vi "Module Init.vi"(8 "error in (no error)":errorcluster, 11 "GUI Manager Module in":refnum<class "GUI Manager Module.lvclass">) -> (0 "error out":errorcluster, 3 "GUI Manager Module out":refnum<class "GUI Manager Module.lvclass">)   [LabVIEW 2020, in "VolatusGUI.lvlib" / "GUI Manager Module.lvclass"]
uses:
  GUI Manager Module.lvclass
  C:/dev/lv20CE/relink/lv-volatus/Volatus/Module/Module.lvclass
  GUI Manager Module.lvclass/GUI Manager Module.ctl
  Volatus/Module/Module.lvclass
  lv-userprefs/User Prefs/PrefsDB/PrefsDB.lvclass
  lv-userprefs/User Prefs/Pref Group/Pref Group.lvclass
  C:/dev/lv20CE/relink/lv-volatus/VolatusGUI/GUI Manager Module/GUI Manager Module.lvclass
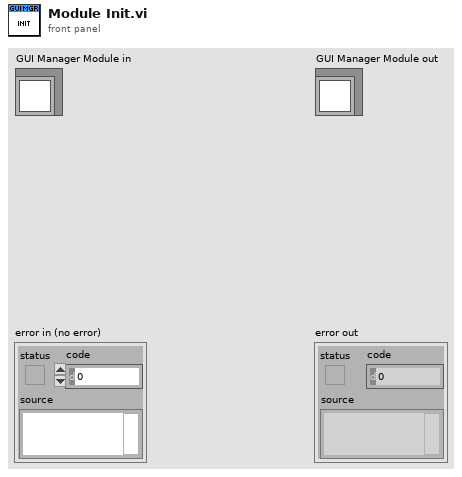
[diagram p1: front panel]
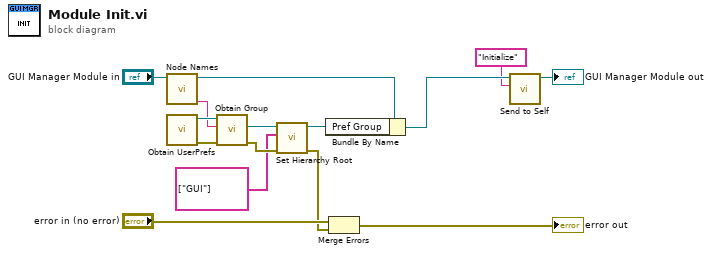
[diagram p0: block diagram]
diagram:
  n1 = call "Node Names.vi"("Module in"="GUI Manager Module in") -> ("Node"=w9:string, "Module out"=w11:refnum<class "GUI Manager Module.lvclass">)  [unwired: 6 in, 3 out]
  n2 = call "Obtain UserPrefs.vi"() -> ("error out"=w14:errorcluster, "PrefsDB out"=w10:refnum<class "PrefsDB.lvclass">)  [unwired: 10 in]
  n3 = call "Obtain Group.vi"("error in (no error)"=w14, "Group"=w9, "PrefsDB in"=w10) -> ("error out"=w15:errorcluster, "Pref Group"=w8:refnum<class "Pref Group.lvclass">)  [unwired: 6 in, 1 out]
  n4 = call "Set Hierarchy Root.vi"("error in (no error)"=w15, "Hierarchy Root"=string[] ["GUI"], "Pref Group in"=w8) -> ("error out"=w3:errorcluster, "Pref Group out"=w5:refnum<class "Pref Group.lvclass">)  [unwired: 7 in]
  n5 = Bundle By Name(cluster=w11, "Pref Group"=w5) -> (w6:refnum<class "GUI Manager Module.lvclass">)
  n6 = Merge Errors("error in (no error)", w3) -> (→"error out":errorcluster)
  n7 = call "Send to Self.vi"("Message ID"="Initialize", "Module in"=w6) -> ("Module out"=→"GUI Manager Module out":refnum<class "GUI Manager Module.lvclass">)  [unwired: 8 in, 1 out]
